vi "sub_save_lotlong.vi"(10 "lat-long":string, 11 "file path":path) -> ()   [LabVIEW 2019]
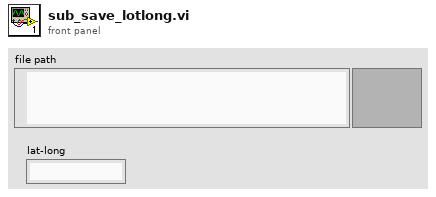
[diagram p1: front panel]
types:
  T1 = enum16{"open", "replace", "create", "open or create", "replace or create", "replace or create with confirmation"}
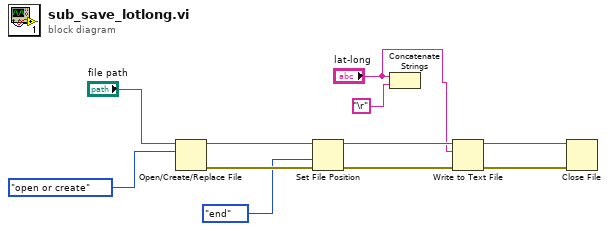
[diagram p0: block diagram]
diagram:
  n1 = Open/Create/Replace File(file path (use dialog)="file path", operation (0:open)=T1."open or create") -> (refnum out=w6:refnum<file>, error out=w5:errorcluster)  [unwired: 4 in, 1 out]
  n2 = Set File Position(refnum=w6, from (0:start)=enum16{"start", "end", "current"}."end", error in=w5) -> (refnum out=w4:refnum<file>, error out=w3:errorcluster)  [unwired: 1 in]
  n3 = Concatenate Strings("lat-long", "\r") -> ()  [unwired: 1 out]
  n4 = Write to Text File(file (use dialog)=w4, text="lat-long", error in=w3) -> (refnum out=w10:refnum<file>, error out=w11:errorcluster)  [unwired: 1 in, 1 out]
  n5 = Close File(refnum=w10, error in=w11) -> ()  [unwired: 2 out]
